vi "Wait for Data.vi"(8 "error in (no error)":errorcluster, 11 "Instrument Recorder in":refnum<class "Instrument Recorder.lvclass">) -> (0 "error out":errorcluster, 3 "Instrument Recorder out":refnum<class "Instrument Recorder.lvclass">)   [LabVIEW 2015, in "Instrument Recorder.lvclass"]
uses:
  Instrument Recorder.lvclass
  Measure Object/Measure Object.lvclass/Measure Object.ctl
  Results/Acquired Result/Acquired Result.lvclass/Acquired Result.ctl
  <vilib>/ActorFramework/Actor/Actor.lvclass/Actor.ctl
  <vilib>/ActorFramework/Message Enqueuer/Message Enqueuer.lvclass/Message Enqueuer.ctl
  Instrument Recorder.lvclass/Instrument Recorder.ctl
  Measure Object/Read Reply to.vi
  Measure Object/Read Name.vi
  Results/Acquired Result/Write Sender.vi
  Results/Acquired Result/Read Finished.vi
  <vilib>/ActorFramework/Message Enqueuer/Init from Existing Queue.vi
  <vilib>/ActorFramework/Time-Delayed Send Message/Time-Delayed Send Message.vi
  Measure Object Messages/Result Reply Msg/Result Reply Msg.lvclass
  <vilib>/ActorFramework/Message Enqueuer/Message Enqueuer.lvclass
  Pulse Recorders/Pulse Recorder Messages/Wait for Data Msg/Wait for Data Msg.lvclass
  <vilib>/ActorFramework/Actor/Actor.lvclass
  Results/Acquired Result/Acquired Result.lvclass
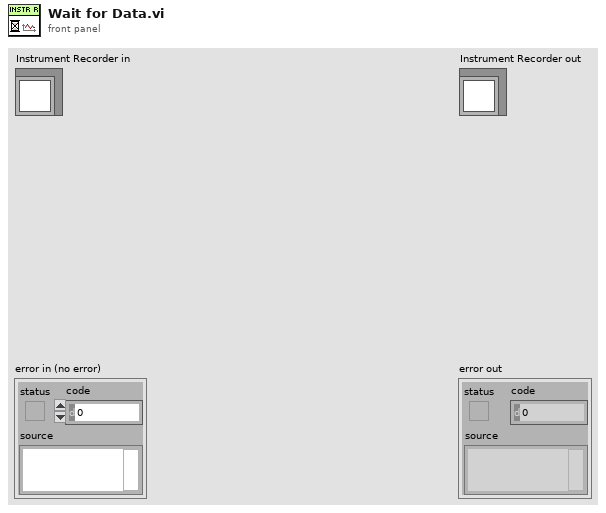
[diagram p1: front panel]
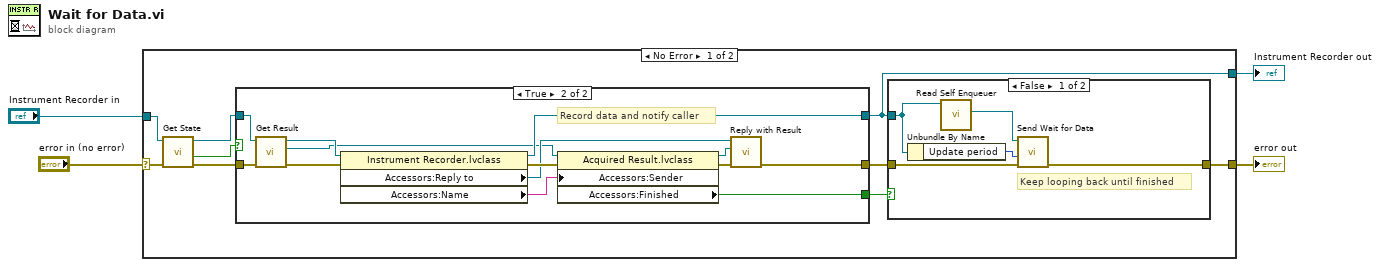
[diagram p0: block diagram]
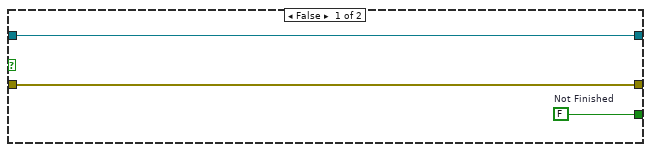
[diagram p3: hidden frame]
diagram:
  n1 = case shown="No Error" "error in (no error)" {
    selector: "error in (no error)" -> [w13 w37]
    tunnel: [w5 w37] -> w3
    tunnel: [w7 w36] -> w1
    tunnel: "Instrument Recorder in" -> [w11 w36]
    frame No Error {
      n2 = call-dynamic "Get State.vi"("error in (no error)"=w13, "Pulse Controller in"=w11) -> ("error out"=w12:errorcluster, "Data ready"=w9:bool, "Pulse Controller out"=w10:refnum<class "Instrument Recorder.lvclass">)  [unwired: 6 in, 1 out]
      n3 = case shown="True" w9 {
        tunnel: w10 -> [w22 w35]
        tunnel: w12 -> [w21 w33]
        tunnel: [w21 w26] -> w6
        tunnel: [w22 w32] -> w7
        tunnel: [w20 w24] -> w8
        frame False {
          w20 = FALSE  # Not Finished
        }
        frame True {
          # "Record data and notify caller"
          n4 = call-dynamic "Get Result.vi"("error in (no error)"=w33, "Instrument Recorder in"=w35) -> ("error out"=w23:errorcluster, "Result"=w25:refnum<class "Acquired Result.lvclass">, "Instrument Recorder out"=w34:refnum<class "Instrument Recorder.lvclass">)  [unwired: 7 in]
          n5 = property class="Instrument Recorder.lvclass"(reference=w34, error in=w23) -> (reference out=w32:refnum<class "Instrument Recorder.lvclass">, error out=w31:errorcluster, "Accessors:Reply to"=w29:refnum<class "Result Reply Msg.lvclass">, "Accessors:Name"=w30:string)
          n6 = property class="Acquired Result.lvclass"(reference=w25, error in=w31, "Accessors:Sender"=w30) -> (reference out=w28:refnum<class "Acquired Result.lvclass">, error out=w27:errorcluster, "Accessors:Finished"=w24:bool)
          n7 = call-dynamic "Reply with Result.vi"("error in (no error)"=w27, "Result"=w28, "Result Reply Msg in"=w29) -> ("error out"=w26:errorcluster)  [unwired: 7 in, 1 out]
        }
      }
      n8 = case shown="False" w8 {
        tunnel: w7 -> [w14 _]
        tunnel: w6 -> [w16 w19]
        tunnel: [w15 w19] -> w5
        frame False {
          # "Keep looping back until finished"
          n9 = Unbundle By Name(w14) -> ("Update period"=w17:i32)
          n10 = call <vilib>:"Read Self Enqueuer.vi"("Actor"=w14) -> ("Self Enqueuer"=w18:refnum<class "Message Enqueuer.lvclass">)  [unwired: 10 in]
          n11 = call "Send Wait for Data.vi"("error in (no error)"=w16, "Milliseconds To Wait"=w17, "Message Enqueuer"=w18) -> ("error out"=w15:errorcluster)  [unwired: 6 in, 2 out]
        }
        frame True {
        }
      }
    }
    frame Error {
    }
  }
  "error out" <- w3
  "Instrument Recorder out" <- w1
